vi "SerialServer.vi"(5 "Stop Refnum":refnum<vi>, 6 "Local Port":u16=16505, 7 "FPGA VI Reference In":refnum<k20>) -> (3 "FPGA VI Reference Out":refnum<k20>)   [LabVIEW 2015]
panel:
  out "Baud Rate":i32(ring)=1 items=["9600"=1, "19200"=2, "38400"=4, "57600"=8, "115200"=16, "230400"=32, "460800"=64, "921600"=128]
  out "error out":errorcluster
  out "OverRunError":bool
  in  "Flush on Close":bool
  out "UART TX count":u64
  out "UART RX count":u64
  out "TCP Bytes Out":u64
  out "Elements in UART TX Queue":i32
  out "Elements in UART RX Queue":i32
  out "TCP Bytes In":u64
  out "connection ID":refnum<k5>
  out "Connected?":bool
  out "Stopped?":bool caption="BeenStopped?"
  out "Remote Address":string
  out "Remote Port":u16
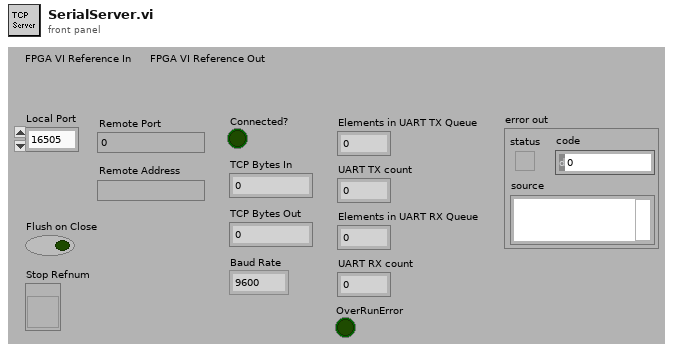
[diagram p1: front panel]
types:
  T1 = enum16{"Standard", "Buffered", "CRLF", "Immediate"}
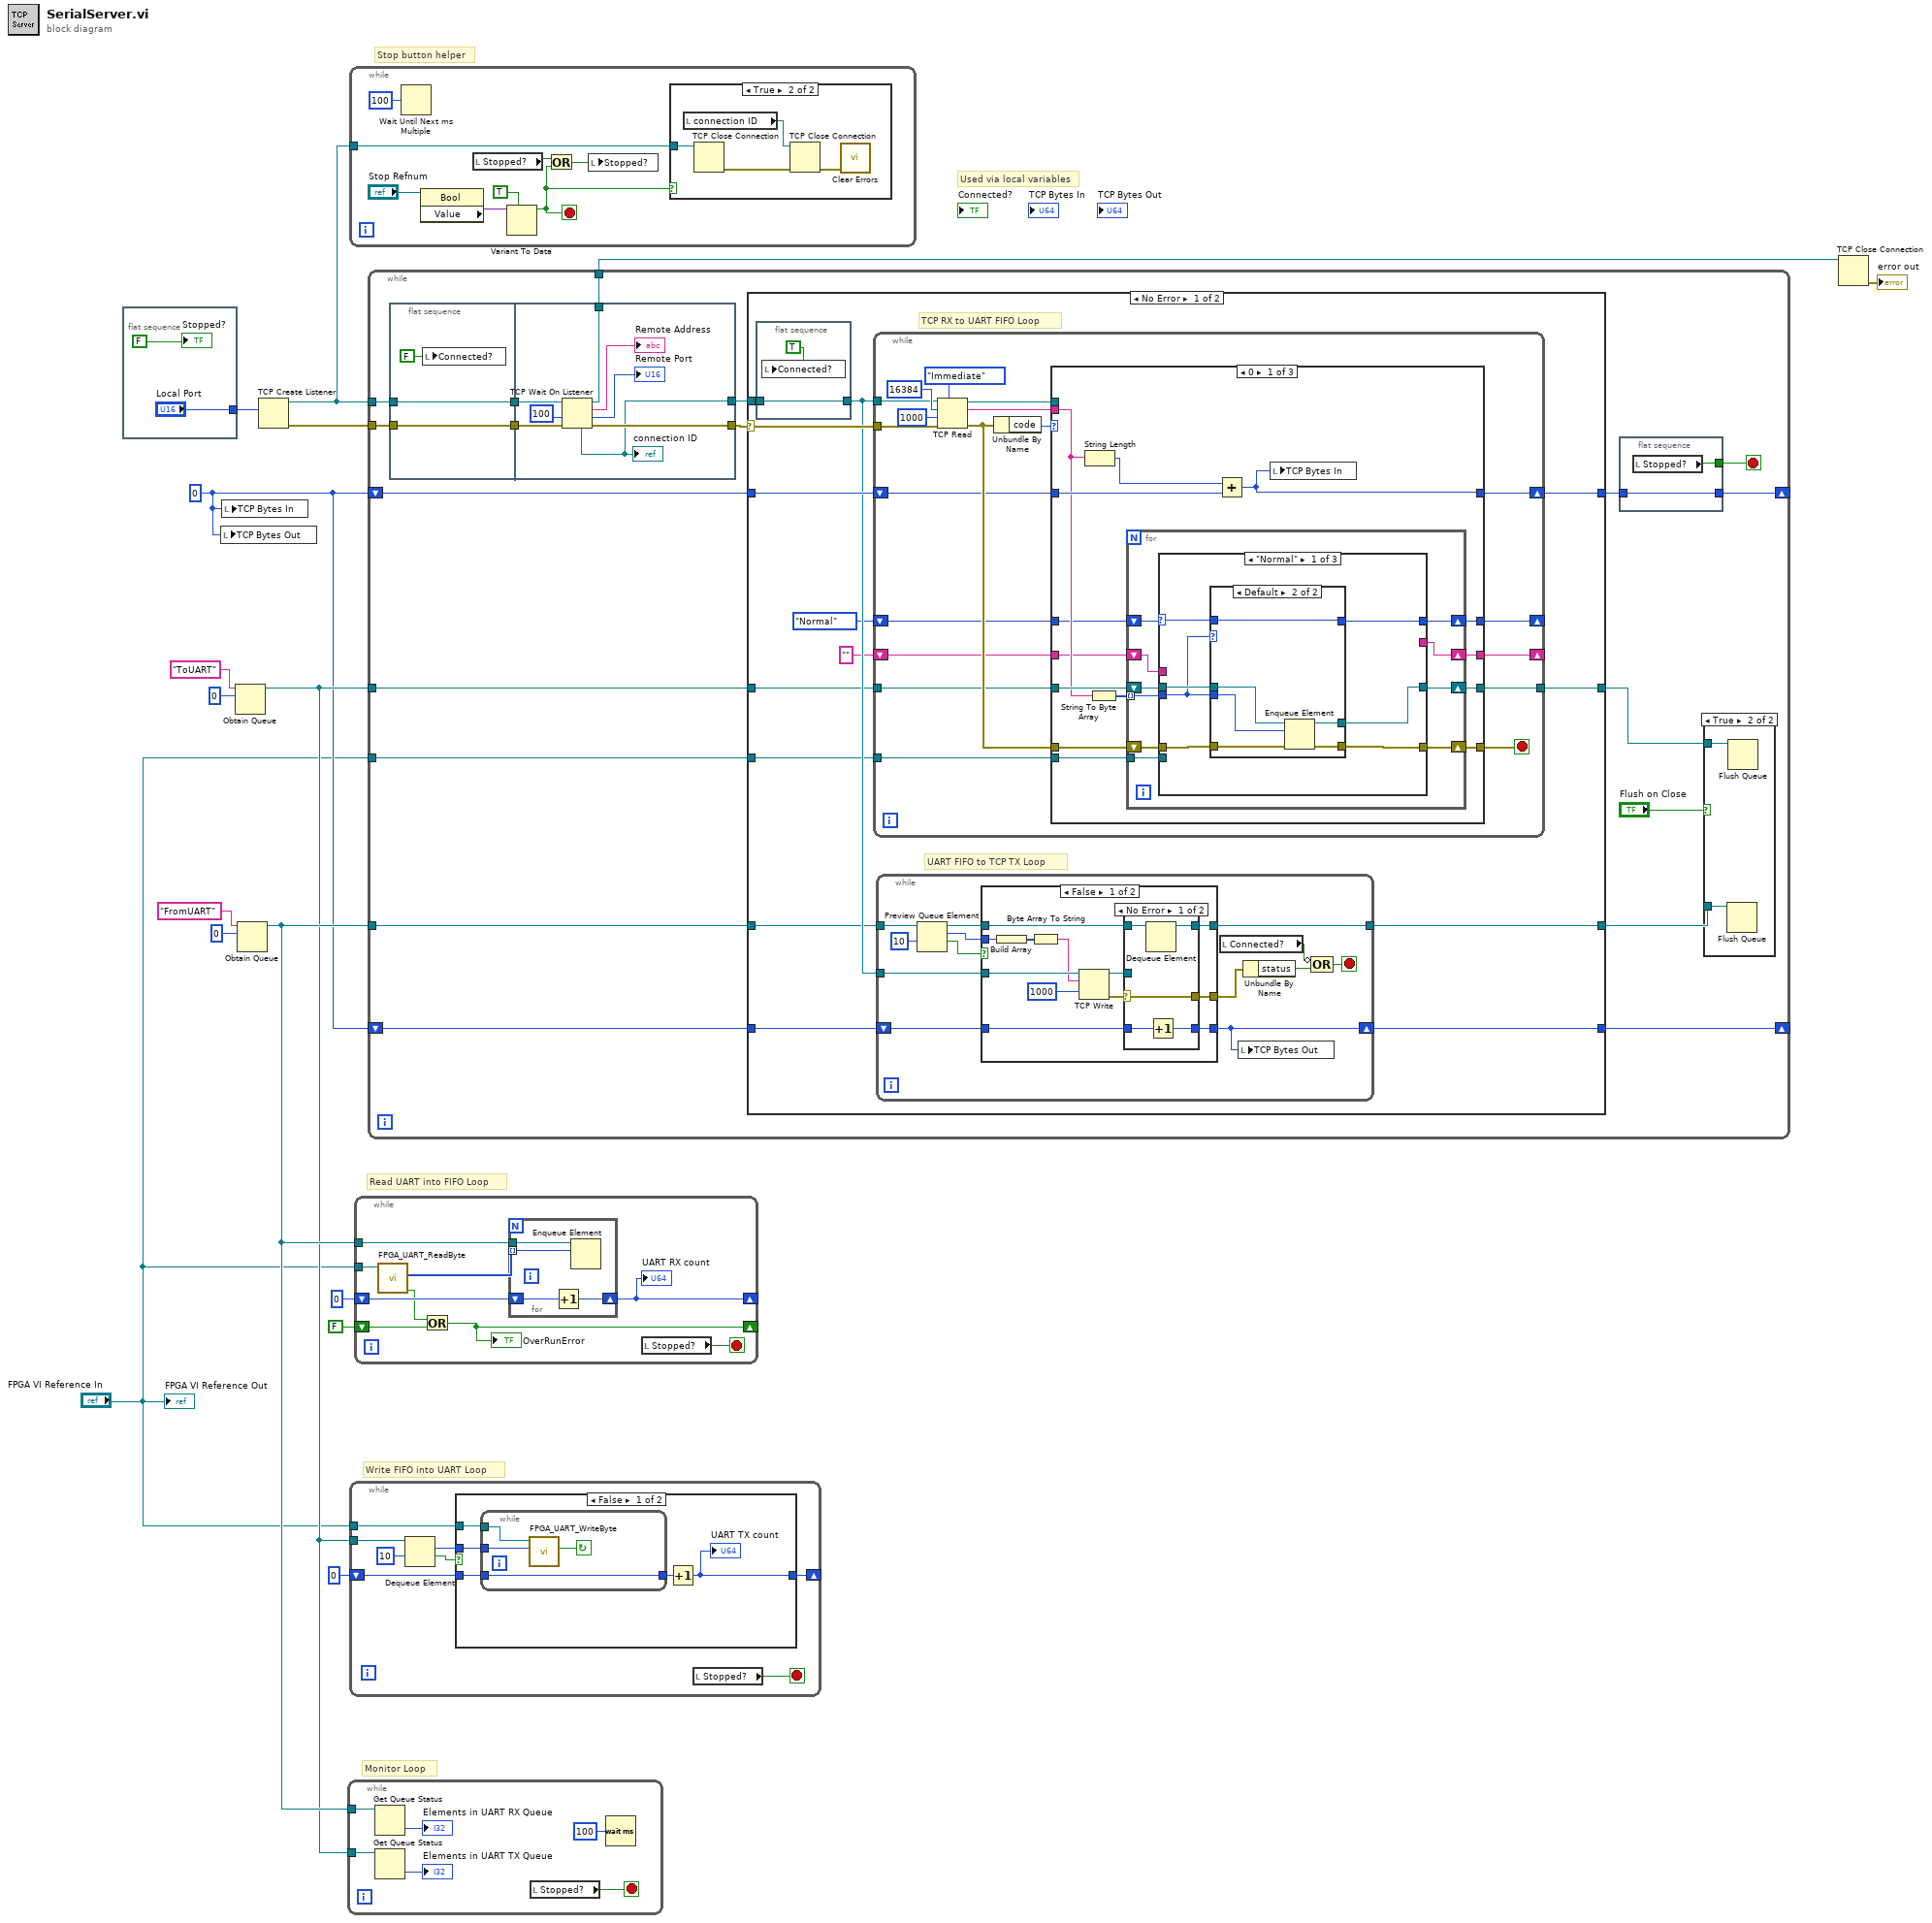
[diagram p0: block diagram]
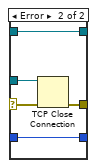
[diagram p5: hidden frame]
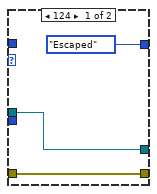
[diagram p7: hidden frame]
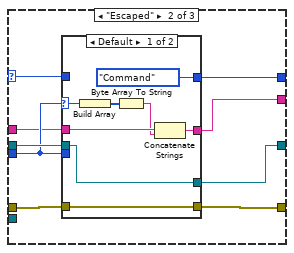
[diagram p8: hidden frame]
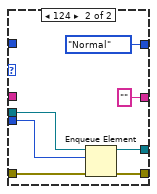
[diagram p9: hidden frame]
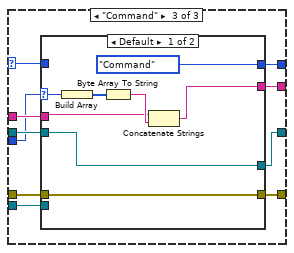
[diagram p10: hidden frame]
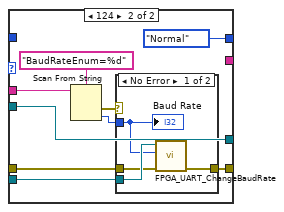
[diagram p11: hidden frame]
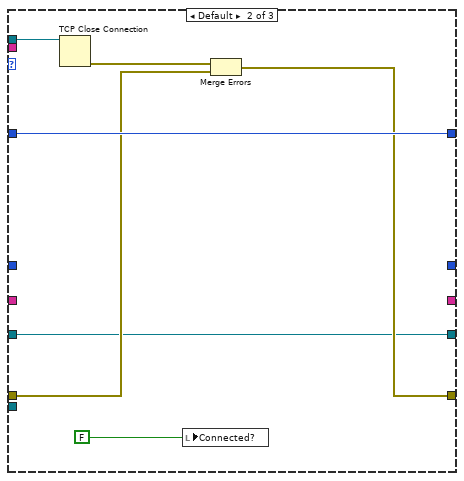
[diagram p13: hidden frame]
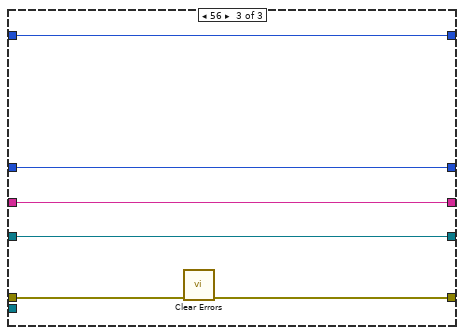
[diagram p14: hidden frame]
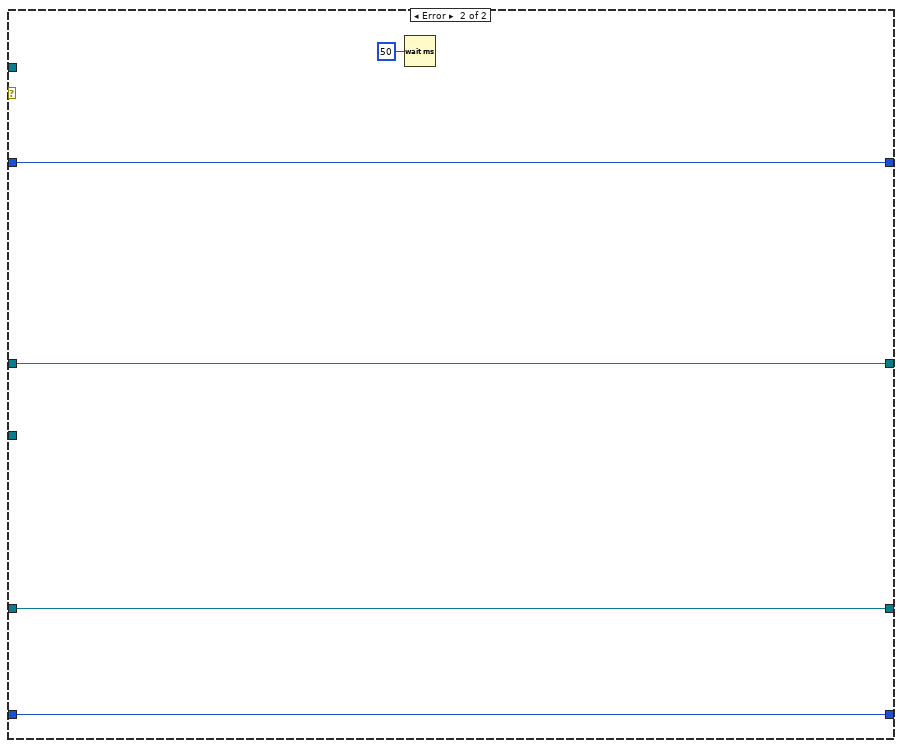
[diagram p15: hidden frame]
diagram:
  w8 = u64 0
  # "Monitor Loop"
  # "Write FIFO into UART Loop"
  # "Read UART into FIFO Loop"
  # "Stop button helper"
  # "Used via local variables"
  n1 = flat-sequence {
    tunnel: ["Local Port"] -> w3
    frame #0 {
      "Stopped?" <- FALSE ("Stopped?")
    }
  }
  n2 = local write "TCP Bytes Out"(w8) -> ()
  n3 = local write "TCP Bytes In"(w8) -> ()
  n4 = Obtain Queue(name (unnamed)="ToUART", element data type=u8 0) -> (queue out=w9:refnum<queue>)  [unwired: 3 in, 2 out]
  n5 = Obtain Queue(name (unnamed)="FromUART", element data type=u8 0) -> (queue out=w10:refnum<queue>)  [unwired: 3 in, 2 out]
  n6 = TCP Create Listener(10:w3) -> (0:w16:errorcluster, 3:w15:refnum<k5>)  [unwired: 1 in, 4 out]
  n7 = while {
    tunnel: w10 -> [w22]
    tunnel: w9 -> [w20]
    stop <- w24 stop-if-true
    n8 = Get Queue Status(queue=w22) -> (# elements in queue=→"Elements in UART RX Queue":i32)  [unwired: 1 in, 8 out]
    n9 = Get Queue Status(queue=w20) -> (# elements in queue=→"Elements in UART TX Queue":i32)  [unwired: 1 in, 8 out]
    n10 = local read "Stopped?"() -> (w24:bool)
    n11 = Wait (ms)(milliseconds to wait=u32 100) -> ()  [unwired: 1 out]
  }
  n12 = while {
    tunnel: w15 -> [w31]
    stop <- w25 stop-if-true
    n13 = Wait Until Next ms Multiple(millisecond multiple=u32 100) -> ()  [unwired: 1 out]
    n14 = property class="Bool"(reference="Stop Refnum") -> ("Value"=w30:variant)  [unwired: 1 in, 2 out]
    n15 = local read "Stopped?"() -> (w26:bool)
    n16 = Variant To Data(type=TRUE ("stop"), Variant=w30) -> (data=w25:bool)  [unwired: 1 in, 1 out]
    n17 = Or(x=w26, y=w25) -> (x .or. y?=w27:bool)
    n18 = local write "Stopped?"(w27) -> ()
    n19 = case shown="True" w25 {
      tunnel: w31 -> [_ w33]
      frame False {
      }
      frame True {
        n20 = local read "connection ID"() -> (w35:refnum<k5>)
        n21 = TCP Close Connection(connection ID=w33) -> (error out=w34:errorcluster)  [unwired: 1 in, 2 out]
        n22 = TCP Close Connection(connection ID=w35, error in (no error)=w34) -> (error out=w36:errorcluster)  [unwired: 2 out]
        n23 = call <vilib>:"Clear Errors.vi"("error in (no error)"=w36) -> ()  [unwired: 1 in, 6 out]
      }
    }
  }
  n24 = while {
    tunnel: w9 -> [w44]
    shift-right: [w38] -> _
    shift-left: u64 0 -> [w39]
    tunnel: "FPGA VI Reference In" -> [w37]
    stop <- w40 stop-if-true
    n25 = Dequeue Element(queue=w44, timeout in ms (-1)=10) -> (element=w41:u8, timed out?=w42:bool)  [unwired: 1 in, 2 out]
    n26 = case shown="False" w42 {
      tunnel: w41 -> [w49 _]
      tunnel: w39 -> [w48 w54]
      tunnel: [w46 w54] -> w38
      tunnel: w37 -> [w45 _]
      frame False {
        n27 = while {
          tunnel: w49 -> [w52]
          tunnel: w48 -> [w53]
          tunnel: [w53] -> w47
          tunnel: w45 -> [w50]
          stop <- w51 continue-if-true
          n28 = call "FPGA_UART_WriteByte.vi"("Byte Value"=w52, "FPGA VI Reference In"=w50) -> ("Overflow?"=w51:bool)  [unwired: 2 in, 6 out]
        }
        n29 = Increment(x=w47) -> (x+1=w46:u64)
        "UART TX count" <- w46
      }
      frame True {
      }
    }
    n30 = local read "Stopped?"() -> (w40:bool)
  }
  n31 = while {
    tunnel: w10 -> [w62]
    shift-right: [w60] -> _
    shift-left: u64 0 -> [w61]
    tunnel: "FPGA VI Reference In" -> [w55]
    shift-right: [w56] -> _
    shift-left: FALSE -> [w57]
    stop <- w63 stop-if-true
    n32 = call "FPGA_UART_ReadByte.vi"("FPGA VI Reference In"=w55) -> ("OverRunError"=w58:bool, "Bytes"=w59:u8[])  [unwired: 9 out]
    n33 = Or(x=w58, y=w57) -> (x .or. y?=w56:bool)
    "OverRunError" <- w56
    n34 = for {
      tunnel: w62 -> [w67]
      tunnel: w59 -> [w64] mode=indexing
      shift-right: [w65] -> w60
      shift-left: w61 -> [w66]
      n35 = Increment(x=w66) -> (x+1=w65:u64)
      n36 = Enqueue Element(queue=w67, element=w64) -> ()  [unwired: 1 in, 4 out]
    }
    "UART RX count" <- w60
    n37 = local read "Stopped?"() -> (w63:bool)
  }
  n38 = while {
    tunnel: w15 -> [w85]
    tunnel: w16 -> [w86]
    shift-right: [w79] -> _
    shift-left: w8 -> [w81]
    tunnel: w9 -> [w78]
    tunnel: w10 -> [w75]
    shift-right: [w73] -> _
    shift-left: w8 -> [w74]
    tunnel: [w69] -> w5
    tunnel: "FPGA VI Reference In" -> [w68]
    stop <- w82 stop-if-true
    n39 = flat-sequence {
      tunnel: w85 -> [w90]
      tunnel: w86 -> [w91]
      tunnel: [w91] -> w77
      tunnel: [w90] -> w76
      tunnel: w77 -> [w97]
      tunnel: w76 -> [w96]
      tunnel: [w95] -> w84
      tunnel: [w92] -> w83
      tunnel: [w93] -> w69
      frame #0 {
        n40 = local write "Connected?"(FALSE ("Connected?")) -> ()
      }
      frame #1 {
        n41 = TCP Wait On Listener(8:w97, 9:100 ("timeout ms (wait forever: -1)"), 11:w96) -> (0:w95:errorcluster, 1:→"Remote Port":u16, 2:→"Remote Address":string, 3:w93:refnum<k5>, 4:w92:refnum<k5>)  [unwired: 1 in]
        "connection ID" <- w92
      }
    }
    n42 = case shown="No Error" w84 {
      selector: w84 -> [w113 _]
      tunnel: w83 -> [w112 _]
      tunnel: w81 -> [w115 w287]
      tunnel: [w114 w287] -> w80
      tunnel: w78 -> [w107 w284]
      tunnel: w75 -> [w108 w285]
      tunnel: w74 -> [w110 w286]
      tunnel: [w109 w286] -> w73
      tunnel: [w106 w284] -> w72
      tunnel: [w105 w285] -> w71
      tunnel: w68 -> [w103 _]
      frame No Error {
        # "UART FIFO to TCP TX Loop"
        # "TCP RX to UART FIFO Loop"
        n43 = flat-sequence {
          tunnel: w112 -> [w153]
          tunnel: [w153] -> w111
          frame #0 {
            n44 = local write "Connected?"(TRUE ("Connected?")) -> ()
          }
        }
        n45 = while {
          tunnel: w113 -> [w166]
          shift-right: [w163] -> w114
          shift-left: w115 -> [w164]
          tunnel: w107 -> [w162]
          tunnel: w111 -> [w161]
          tunnel: [w160] -> w106
          shift-right: [w155] -> _
          shift-left: "" -> [w159]
          shift-right: [w156] -> _
          shift-left: enum16{"Normal", "Escaped", "Command"}."Normal" -> [w158]
          tunnel: w103 -> [w157]
          stop <- w167 stop-if-true
          n46 = TCP Read(connection ID=w161, bytes to read=16384, error in (no error)=w166, 7:T1."Immediate" ("mode (standard)"), 9:1000 ("timeout ms (25000)")) -> (connection ID out=w169:refnum<k5>, data out=w168:string, error out=w170:errorcluster)
          n47 = Unbundle By Name(w170) -> ("code"=w171:i32)
          n48 = case shown="0" w171 {
            tunnel: w170 -> [w181 w274 w282]
            tunnel: w169 -> [_ w275 _]
            tunnel: w168 -> [w183 _ _]
            tunnel: [w180 w272 w281] -> w167
            tunnel: w164 -> [w187 w276 w280]
            tunnel: [w186 w276 w280] -> w163
            tunnel: w162 -> [w185 w270 w279]
            tunnel: [w179 w270 w279] -> w160
            tunnel: w159 -> [w178 _ w277]
            tunnel: w158 -> [w177 _ w278]
            tunnel: w157 -> [w176 _ _]
            tunnel: [w175 _ w278] -> w156
            tunnel: [w174 _ w277] -> w155
            frame 0 {
              n49 = String Length(string=w183) -> (length=w184:i32)
              n50 = String To Byte Array(string=w183) -> (unsigned byte array=w182:u8[])
              n51 = for {
                tunnel: w182 -> [w193] mode=indexing
                shift-right: [w195] -> w180
                shift-left: w181 -> [w196]
                shift-right: [w194] -> w179
                shift-left: w185 -> [w197]
                shift-right: [w188] -> w174
                shift-left: w178 -> [w190]
                shift-right: [w191] -> w175
                shift-left: w177 -> [w192]
                tunnel: w176 -> [w189]
                n52 = case shown="\"Normal\"" w192 {
                  selector: w192 -> [w198 w216 w242]
                  tunnel: w197 -> [w204 w222 w247]
                  tunnel: w193 -> [w200 w218 w239]
                  tunnel: w196 -> [w203 w221 w246]
                  tunnel: [w202 w220 w245] -> w195
                  tunnel: [w201 w219 w244] -> w194
                  tunnel: [w199 w217 w243] -> w191
                  tunnel: w190 -> [_ w215 w241]
                  tunnel: w189 -> [_ _ w240]
                  tunnel: [_ w214 w238] -> w188
                  frame "Normal" {
                    n53 = case shown="Default" w200 {
                      tunnel: w204 -> [w206 w213]
                      tunnel: w200 -> [_ w212]
                      tunnel: w203 -> [w205 w211]
                      tunnel: [w205 w210] -> w202
                      tunnel: [w206 w209] -> w201
                      tunnel: [enum16{"Normal", "Escaped", "Command"}."Escaped" w208] -> w199
                      tunnel: w198 -> [_ w208]
                      frame 124 {
                      }
                      frame Default {
                        n54 = Enqueue Element(queue=w213, element=w212, error in (no error)=w211) -> (queue out=w209:refnum<queue>, error out=w210:errorcluster)  [unwired: 2 out]
                      }
                    }
                  }
                  frame "Escaped" {
                    n55 = case shown="Default" w218 {
                      selector: w218 -> [w227 _]
                      tunnel: w222 -> [w229 w237]
                      tunnel: w218 -> [_ w236]
                      tunnel: w221 -> [w228 w235]
                      tunnel: [w228 w234] -> w220
                      tunnel: [w229 w233] -> w219
                      tunnel: [enum16{"Normal", "Escaped", "Command"}."Command" enum16{"Normal", "Escaped", "Command"}."Normal"] -> w217
                      tunnel: w216 -> [_ _]
                      tunnel: w215 -> [w225 _]
                      tunnel: [w223 ""] -> w214
                      frame Default {
                        n56 = Build Array(w227) -> (w226:u8[])
                        n57 = Byte Array To String(unsigned byte array=w226) -> (string=w224:string)
                        n58 = Concatenate Strings(w225, w224) -> (w223:string)
                      }
                      frame 124 {
                        n59 = Enqueue Element(queue=w237, element=w236, error in (no error)=w235) -> (queue out=w233:refnum<queue>, error out=w234:errorcluster)  [unwired: 2 out]
                      }
                    }
                  }
                  frame "Command" {
                    n60 = case shown="Default" w239 {
                      selector: w239 -> [w252 _]
                      tunnel: w247 -> [w254 w263]
                      tunnel: w246 -> [w253 w258]
                      tunnel: [w253 w257] -> w245
                      tunnel: [w254 w263] -> w244
                      tunnel: [enum16{"Normal", "Escaped", "Command"}."Command" enum16{"Normal", "Escaped", "Command"}."Normal"] -> w243
                      tunnel: w242 -> [_ _]
                      tunnel: w241 -> [w249 w256]
                      tunnel: w240 -> [_ w259]
                      tunnel: [w248 _] -> w238
                      frame Default {
                        n61 = Build Array(w252) -> (w251:u8[])
                        n62 = Byte Array To String(unsigned byte array=w251) -> (string=w250:string)
                        n63 = Concatenate Strings(w249, w250) -> (w248:string)
                      }
                      frame 124 {
                        n64 = Scan From String(format string="BaudRateEnum=%d", input string=w256) -> (error out=w261:errorcluster, output 1=w260:i32)  [unwired: 3 in, 2 out]
                        n65 = case shown="No Error" w261 {
                          tunnel: w260 -> [w265 _]
                          tunnel: w259 -> [w268 _]
                          tunnel: w258 -> [w267 w269]
                          tunnel: [w266 w269] -> w257
                          frame No Error {
                            n66 = call "FPGA_UART_ChangeBaudRate.vi"("error  in"=w267, "Baud Rate Enum"=w265, "FPGA VI Reference In"=w268) -> ("error out"=w266:errorcluster)  [unwired: 6 in, 1 out]
                            "Baud Rate" <- w265
                          }
                          frame Error {
                          }
                        }
                      }
                    }
                  }
                }
              }
              n67 = Add(x=w184, y=w187) -> (x+y=w186:u64)
              n68 = local write "TCP Bytes In"(w186) -> ()
            }
            frame Default {
              n69 = TCP Close Connection(connection ID=w275) -> (error out=w273:errorcluster)  [unwired: 1 in, 2 out]
              n70 = local write "Connected?"(FALSE ("Connected?")) -> ()
              n71 = Merge Errors(w273, w274) -> (w272:errorcluster)
            }
            frame 56 {
              n72 = call <vilib>:"Clear Errors.vi"("error in (no error)"=w282) -> ("error out"=w281:errorcluster)  [unwired: 1 in, 5 out]
            }
          }
        }
        n73 = while {
          tunnel: w111 -> [w124]
          tunnel: w108 -> [w127]
          tunnel: [w116] -> w105
          shift-right: [w120] -> w109
          shift-left: w110 -> [w122]
          stop <- w117 stop-if-true
          n74 = Preview Queue Element(queue=w127, timeout in ms (-1)=10) -> (queue out=w121:refnum<queue>, element=w125:u8, timed out?=w126:bool)  [unwired: 1 in, 1 out]
          n75 = case shown="False" w126 {
            tunnel: w125 -> [w139 _]
            tunnel: w124 -> [w140 _]
            tunnel: [w134 _] -> w123
            tunnel: w122 -> [w131 w152]
            tunnel: [w130 w152] -> w120
            tunnel: w121 -> [w132 w151]
            tunnel: [w129 w151] -> w116
            frame False {
              n76 = Build Array(w139) -> (w138:u8[])
              n77 = Byte Array To String(unsigned byte array=w138) -> (string=w137:string)
              n78 = TCP Write(connection ID=w140, data in=w137, 9:1000 ("timeout ms (25000)")) -> (connection ID out=w133:refnum<k5>, error out=w135:errorcluster)  [unwired: 1 in, 1 out]
              n79 = case shown="No Error" w135 {
                selector: w135 -> [w145 w149]
                tunnel: [w145 w148] -> w134
                tunnel: w133 -> [_ w150]
                tunnel: w132 -> [w144 w146]
                tunnel: w131 -> [w143 w147]
                tunnel: [w142 w147] -> w130
                tunnel: [w141 w146] -> w129
                frame No Error {
                  n80 = Dequeue Element(queue=w144) -> (queue out=w141:refnum<queue>)  [unwired: 2 in, 3 out]
                  n81 = Increment(x=w143) -> (x+1=w142:u64)
                }
                frame Error {
                  n82 = TCP Close Connection(connection ID=w150, error in (no error)=w149) -> (error out=w148:errorcluster)  [unwired: 2 out]
                }
              }
            }
            frame True {
            }
          }
          n83 = local read "Connected?"() -> (w119:bool)
          n84 = local write "TCP Bytes Out"(w120) -> ()
          n85 = Unbundle By Name(w123) -> ("status"=w118:bool)
          n86 = Compound Arithmetic op=OR(invert w119, w118) -> (w117:bool)
        }
      }
      frame Error {
        n87 = Wait (ms)(milliseconds to wait=u32 50) -> ()  [unwired: 1 out]
      }
    }
    n88 = flat-sequence {
      tunnel: [w101] -> w82
      tunnel: w80 -> [w100]
      tunnel: [w100] -> w79
      frame #0 {
        n89 = local read "Stopped?"() -> (w101:bool)
      }
    }
    n90 = case shown="True" "Flush on Close" {
      tunnel: w72 -> [_ w88]
      tunnel: w71 -> [_ w87]
      frame False {
      }
      frame True {
        n91 = Flush Queue(queue=w87) -> ()  [unwired: 1 in, 3 out]
        n92 = Flush Queue(queue=w88) -> ()  [unwired: 1 in, 3 out]
      }
    }
  }
  n93 = TCP Close Connection(connection ID=w5) -> (error out=→"error out":errorcluster)  [unwired: 2 in, 1 out]
  "FPGA VI Reference Out" <- "FPGA VI Reference In"
